vi "Helper - 0-360 angle subtraction, addition.vi"(8 "y":dbl, 11 "x":dbl) -> (0 "x + y":dbl, 3 "x - y":T1)   [LabVIEW 2011]
doc: "Takes in two angles and adds and subtracts them, then makes sure that the outputs are both in the 0 to 360 range."
uses:
  2 Typedefs/apparent wind direction.ctl
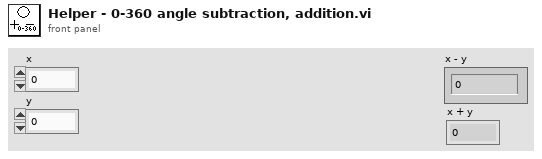
[diagram p1: front panel]
types:
  T1 = typedef "apparent wind direction.ctl" = dbl
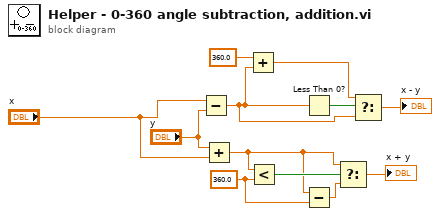
[diagram p0: block diagram]
diagram:
  w1 = 360.0 ("y")
  n1 = Subtract(x="x", y="y") -> (x-y=w11:dbl)
  n2 = Add(x="y", y="x") -> (x+y=w6:dbl)
  n3 = Add(x=T1 360.0, y=w11) -> (x+y=w9:T1)
  n4 = Less?(x=w6, y=w1) -> (x < y?=w8:bool)
  n5 = Less Than 0?(x=w11) -> (x < 0?=w12:bool)
  n6 = Subtract(x=w6, y=w1) -> (x-y=w7:dbl)
  n7 = Select(t=w6, s=w8, f=w7) -> (s? t:f=→"x + y":dbl)
  n8 = Select(t=w9, s=w12, f=w11) -> (s? t:f=→"x - y":T1)
